vi "DHT Pressure 2016.vi"(0 "Sensor Cluster":T1, 1 "DHT Pressure Offset":dbl format="%.2f", 2 "Array in":refnum<k24>[](array[refnum]), 5 "DHT Pressure \nSlope":dbl=24.27199935913086 format="%.2f", 7 "Descriptions":string[](array[string]), 9 "Zero Pressure\n(F = leave as is)":bool) -> (3 "Array out":refnum<k24>[](array[refnum]), 4 "DHT Pressure (ft/H20)":dbl format="%.2f", 6 "DHT Pressure (V)":dbl format="%.2f", 13 "Sensor Cluster out":T1)   [LabVIEW 2016]
uses:
  controls/MCC DAQ Readings.ctl
  C:/Cascade-lv16-64/builds/Waterloo Main Program/cascade/data/ULx_LV.dll
  builds/Waterloo Main Program/cascade/data/ULx_LV.dll
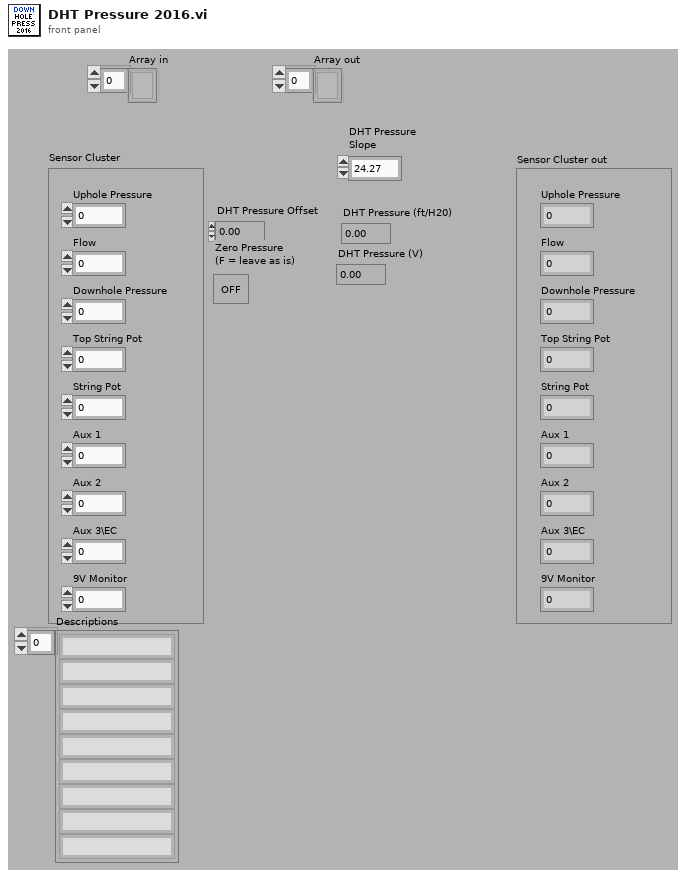
[diagram p1: front panel]
types:
  T1 = typedef "MCC DAQ Readings.ctl" = cluster{"Uphole Pressure":dbl, "Flow":dbl, "Downhole Pressure":dbl, "Top String Pot":dbl, "String Pot":dbl, "Aux 1":dbl, "Aux 2":dbl, "Aux 3\\EC":dbl, "9V Monitor":dbl}
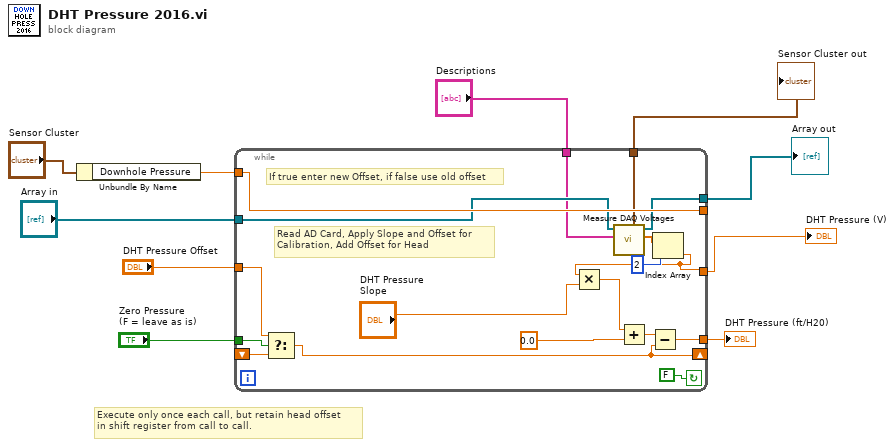
[diagram p0: block diagram]
diagram:
  # "Execute only once each call, but retain head offset \nin shift register from call to call."
  n1 = Unbundle By Name("Sensor Cluster") -> ("Downhole Pressure"=w7:dbl)
  n2 = while {
    tunnel: "Zero Pressure\n(F = leave as is)" -> [w24]
    tunnel: "DHT Pressure Offset" -> [w25]
    shift-left: _ -> [w26]
    shift-right: [w20] -> _
    tunnel: [w23] -> w10
    tunnel: [w19] -> _
    tunnel: w7 -> [w19]
    tunnel: "Array in" -> [w17]
    tunnel: [w16] -> w5
    tunnel: [w15] -> w3
    tunnel: "Descriptions" -> [w13]
    tunnel: [w11] -> w1
    stop <- FALSE continue-if-true
    # "Read AD Card, Apply Slope and Offset for\nCalibration, Add Offset for Head"
    # "If true enter new Offset, if false use old offset"
    n3 = Select(t=w25, s=w24, f=w26) -> (s? t:f=w20:dbl)
    n4 = call "Measure DAQ Voltages.vi"("Descriptions"=w13, "Array in"=w17) -> ("Raw Voltages"=w14:dbl[], "Array out"=w16:refnum<k24>[], "Sensor Cluster"=w15:T1)  [unwired: 6 in, 1 out]
    n5 = Index Array(array=w14, index=2) -> (element=w11:dbl)
    n6 = Multiply(x=w11, y="DHT Pressure \nSlope") -> (x*y=w28:dbl)
    n7 = Add(x=w28, y=0.0 ("Offset")) -> (x+y=w21:dbl)
    n8 = Subtract(x=w21, y=w20) -> (x-y=w23:dbl)
  }
  "DHT Pressure (ft/H20)" <- w10
  "DHT Pressure (V)" <- w1
  "Array out" <- w5
  "Sensor Cluster out" <- w3
